vi "test_AK RS-xxx Get Protocol Type.vi"(8 "error in (no error)":errorcluster, 11 "TestCase in":refnum<class "Instrument Addon Scripting API Protocol Factories Unit Tests.lvclass">) -> (0 "error out":errorcluster, 3 "TestCase out":refnum<class "Instrument Addon Scripting API Protocol Factories Unit Tests.lvclass">)   [LabVIEW 2023, in "Instrument Addon Scripting API Protocol Factories Unit Tests.lvclass"]
uses:
  Instrument Addon Scripting API Protocol Factories Unit Tests.lvclass
  <vilib>/addons/_JKI Toolkits/VI Tester/TestCase.llb/TestCase.lvclass
  Protocol Parent/Types/Protocol Type.ctl
  Protocol Parent/Protocol Parent.lvclass
  AK RS-xxx/AK RS-xxx.lvclass
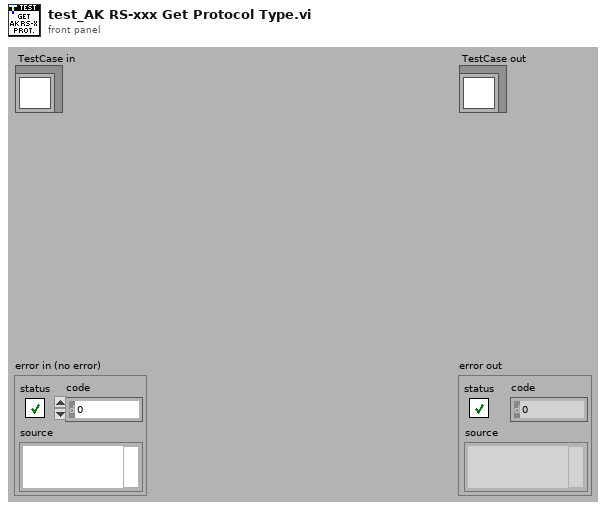
[diagram p1: front panel]
types:
  T1 = typedef "Protocols.lvlib/Protocol Parent.lvclass/Protocol Type.ctl" = enum16{"RS-XXX", "AK RS-XXX", "VISA", "TCPIP", "AK TCPIP", "UDP", "GPIB ConvBox"}
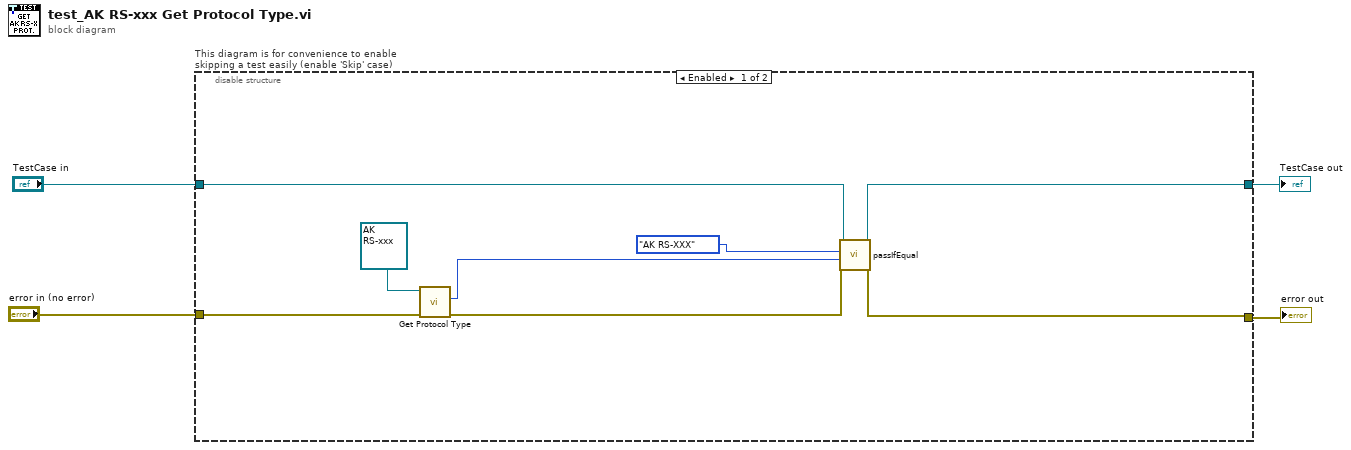
[diagram p0: block diagram]
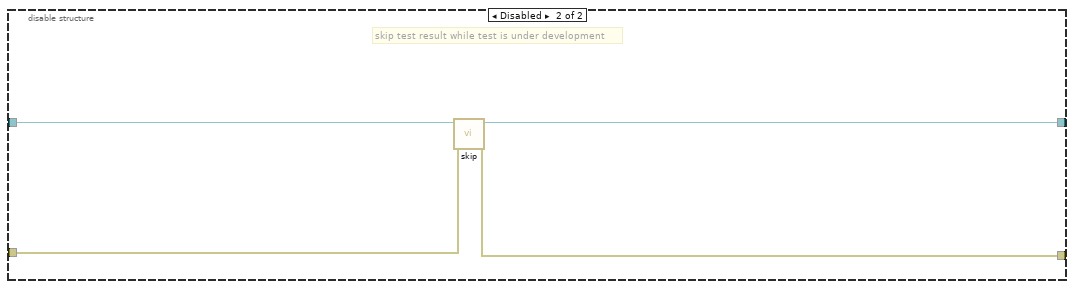
[diagram p2: hidden frame]
diagram:
  n1 = disable-structure "This diagram is for convenience to enable skipping a test easily (enable 'Skip' case)" shown="Enabled" {
    disable-tunnel: "TestCase in" -> [w12 w16]
    disable-tunnel: [w11 w14] -> w1
    disable-tunnel: [w10 w15] -> w3
    disable-tunnel: "error in (no error)" -> [w8 w13]
    frame Enabled {
      n2 = call-dynamic "Get Protocol Type.vi"("error in (no error)"=w8, "AK RS-xxx in"=refnum<class "AK RS-xxx.lvclass"> refnum ("Protocols.lvlib:AK RS-xxx.lvclass")) -> ("error out"=w9:errorcluster, "protocol type"=w7:T1)  [unwired: 7 in, 1 out]
      n3 = call-dynamic "passIfEqual.vi"("error in (no error)"=w9, "y"=w7, "x"=Protocol_Type."AK RS-XXX" ("Protocol Type"), "TestCase in"=w12) -> ("error out"=w10:errorcluster, "TestCase out"=w11:refnum<class "Instrument Addon Scripting API Protocol Factories Unit Tests.lvclass">)  [unwired: 6 in]
    }
    frame Disabled {
      # "skip test result while test is under development"
      n4 = call <vilib>:"skip.vi"("error in (no error)"=w13, "TestCase in"=w16) -> ("error out"=w15:errorcluster, "TestCase out"=w14:refnum<class "Instrument Addon Scripting API Protocol Factories Unit Tests.lvclass">)  [unwired: 8 in]
    }
  }
  "error out" <- w3
  "TestCase out" <- w1
